vi "START command.vi"(8 "Error In":errorcluster, 11 "SerialComm in":refnum<class "SerialComm.lvclass">) -> (0 "Error Out":errorcluster, 3 "SerialComm out":refnum<class "SerialComm.lvclass">)   [LabVIEW 2016, in "SerialComm.lvclass"]
uses:
  SerialComm.lvclass
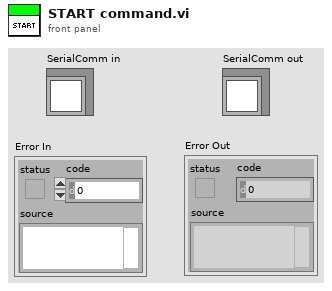
[diagram p1: front panel]
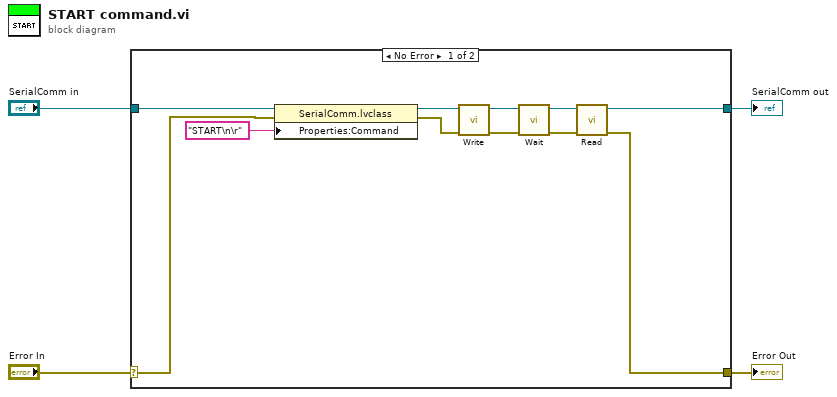
[diagram p0: block diagram]
diagram:
  n1 = case shown="No Error" "Error In" {
    selector: "Error In" -> [w11 w17]
    tunnel: [w5 w17] -> w3
    tunnel: [w8 w16] -> w1
    tunnel: "SerialComm in" -> [w15 w16]
    frame No Error {
      n2 = property class="SerialComm.lvclass"(reference=w15, error in=w11, "Properties:Command"="START\n\r" ("Command")) -> (reference out=w14:refnum<class "SerialComm.lvclass">, error out=w10:errorcluster)
      n3 = call "Write.vi"("Error In"=w10, "SerialComm in"=w14) -> ("Error Out"=w7:errorcluster, "SerialComm out"=w12:refnum<class "SerialComm.lvclass">)  [unwired: 8 in]
      n4 = call "Wait.vi"("Error In"=w7, "SerialComm in"=w12) -> ("Error Out"=w6:errorcluster, "SerialComm out"=w9:refnum<class "SerialComm.lvclass">)  [unwired: 8 in]
      n5 = call "Read.vi"("Error In"=w6, "SerialComm in"=w9) -> ("Error Out"=w5:errorcluster, "SerialComm out"=w8:refnum<class "SerialComm.lvclass">)  [unwired: 8 in]
    }
    frame Error {
    }
  }
  "Error Out" <- w3
  "SerialComm out" <- w1
